vi "oa_Config Scale and Unit for Waterfall Plot.vi"(0 "waterfall plot ref":refnum<vi>, 1 "plot type":T1(ring), 5 "scales":T3 {"Y scale"."multiplier" format="%.2f"; "Y scale"."offset" format="%.2f"; "X scale"."multiplier" format="%.2f"; "X scale"."offset" format="%.2f"}, 7 "unit labels":T2, 9 "spectral map":dbl[][](array[numeric]) format="%.2f", 11 "error in (no error)":errorcluster, 12 "dB on":bool=TRUE) -> (6 "X scale":cluster{"offset":dbl, "multiplier":dbl} {"multiplier" format="%.2f"; "offset" format="%.2f"}, 8 "Y scale":cluster{"offset":dbl, "multiplier":dbl} {"multiplier" format="%.2f"; "offset" format="%.2f"}, 10 "spectral map out":dbl[][](array[numeric]) format="%.2f", 15 "error out":errorcluster)   [LabVIEW 2017]
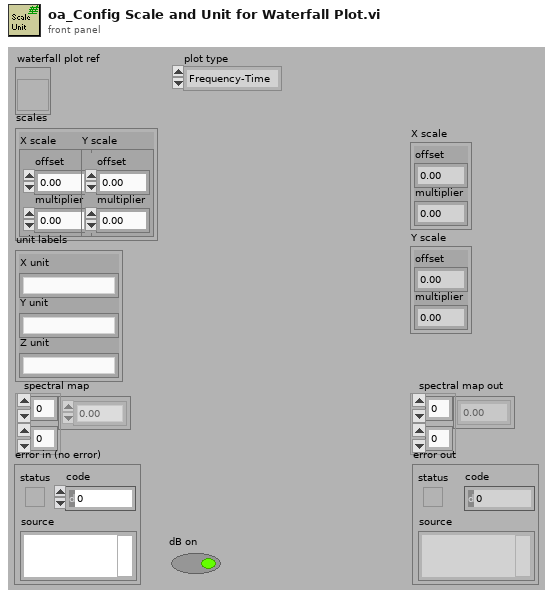
[diagram p1: front panel]
types:
  T1 = enum16{"Frequency-Time", "Time-Frequency", "Order-Time", "Time-Order", "Frequency-RPM", "RPM-Frequency", "Order-RPM", "RPM-Order"}
  T2 = cluster{"X unit":string, "Y unit":string, "Z unit":string}
  T3 = cluster{"X scale":cluster{"offset":dbl, "multiplier":dbl}, "Y scale":cluster{"offset":dbl, "multiplier":dbl}}
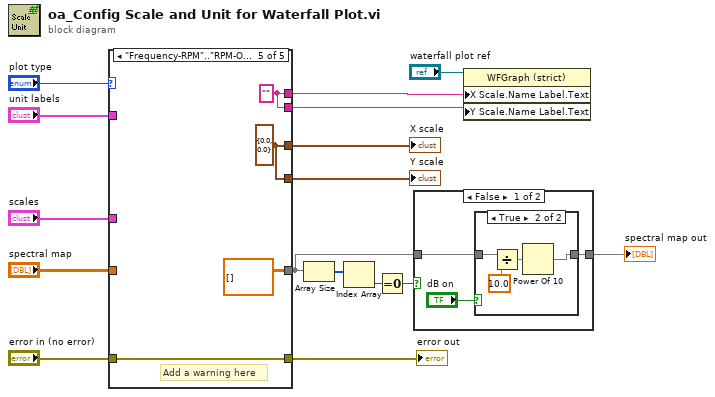
[diagram p0: block diagram]
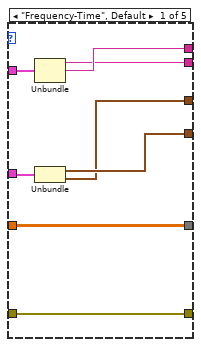
[diagram p4: hidden frame]
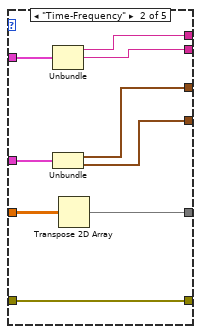
[diagram p5: hidden frame]
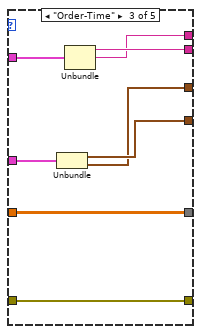
[diagram p6: hidden frame]
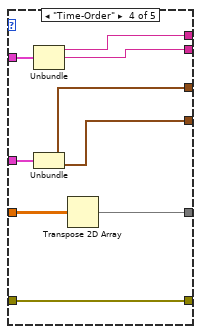
[diagram p7: hidden frame]
diagram:
  n1 = case shown="\"Frequency-RPM\"..\"RPM-Order\"" "plot type" {
    tunnel: "scales" -> [w24 w33 w41 w50 _]
    tunnel: [w23 w31 w40 w49 w53] -> w14
    tunnel: [w22 w32 w39 w48 w53] -> w13
    tunnel: "unit labels" -> [w21 w30 w38 w47 _]
    tunnel: [w20 w29 w36 w46 w54] -> w11
    tunnel: [w19 w28 w37 w45 w54] -> w10
    tunnel: "spectral map" -> [w18 w27 w35 w44 _]
    tunnel: [w18 w26 w35 w43 dbl[][] [] ("spectral map")] -> w2
    tunnel: "error in (no error)" -> [w17 w25 w34 w42 w51]
    tunnel: [w17 w25 w34 w42 w51] -> w6
    frame "Frequency-Time", Default {
      n2 = Unbundle(w21) -> ("X unit"=w19:string, "Y unit"=w20:string)  [unwired: 1 out]
      n3 = Unbundle(w24) -> ("X scale"=w23:cluster{"offset":dbl, "multiplier":dbl}, "Y scale"=w22:cluster{"offset":dbl, "multiplier":dbl})
    }
    frame "Time-Frequency" {
      n4 = Unbundle(w30) -> ("X unit"=w29:string, "Y unit"=w28:string)  [unwired: 1 out]
      n5 = Unbundle(w33) -> ("X scale"=w32:cluster{"offset":dbl, "multiplier":dbl}, "Y scale"=w31:cluster{"offset":dbl, "multiplier":dbl})
      n6 = Transpose 2D Array(2D array=w27) -> (transposed array=w26:dbl[][])
    }
    frame "Order-Time" {
      n7 = Unbundle(w41) -> ("X scale"=w40:cluster{"offset":dbl, "multiplier":dbl}, "Y scale"=w39:cluster{"offset":dbl, "multiplier":dbl})
      n8 = Unbundle(w38) -> ("X unit"=w37:string, "Y unit"=w36:string)  [unwired: 1 out]
    }
    frame "Time-Order" {
      n9 = Unbundle(w47) -> ("X unit"=w46:string, "Y unit"=w45:string)  [unwired: 1 out]
      n10 = Unbundle(w50) -> ("X scale"=w48:cluster{"offset":dbl, "multiplier":dbl}, "Y scale"=w49:cluster{"offset":dbl, "multiplier":dbl})
      n11 = Transpose 2D Array(2D array=w44) -> (transposed array=w43:dbl[][])
    }
    frame "Frequency-RPM".."RPM-Order" {
      w54 = ""
      w53 = cluster{"offset":dbl, "multiplier":dbl} {"offset"=0.0, "multiplier"=0.0}
      # "Add a warning here"
    }
  }
  "X scale" <- w13
  "Y scale" <- w14
  "error out" <- w6
  n12 = Array Size(array=w2) -> (size(s)=w5:i32[])
  n13 = Index Array(array=w5) -> (element=w4:i32)  [unwired: 1 in]
  n14 = Equal To 0?(x=w4) -> (x = 0?=w3:bool)
  n15 = case shown="False" w3 {
    tunnel: w2 -> [w56 w63]
    tunnel: [w55 w63] -> w1
    frame False {
      n16 = case shown="True" "dB on" {
        tunnel: w56 -> [w58 w62]
        tunnel: [w58 w59] -> w55
        frame False {
        }
        frame True {
          n17 = Divide(x=w62, y=10.0) -> (x/y=w60:dbl[][])
          n18 = Power Of 10(x=w60) -> (10^x=w59:dbl[][])
        }
      }
    }
    frame True {
    }
  }
  "spectral map out" <- w1
  n19 = property class="WFGraph (strict)"(reference="waterfall plot ref", "X Scale.Name Label.Text"=w11, "Y Scale.Name Label.Text"=w10) -> ()  [unwired: 1 in, 2 out]
